vi "to_json.vi"(8 "error in":errorcluster, 11 "filterTypes in":refnum<class "filterTypes.lvclass">) -> (0 "error out":errorcluster, 2 "json":string, 3 "filterTypes out":refnum<class "filterTypes.lvclass">, 4 "Not Default":bool)   [LabVIEW 2020, in "nominal types.lvlib" / "channelFilter.lvlib" / "filterTypes.lvclass"]
uses:
  filterTypes.lvclass
  filterTypes.lvclass/filterTypes.ctl
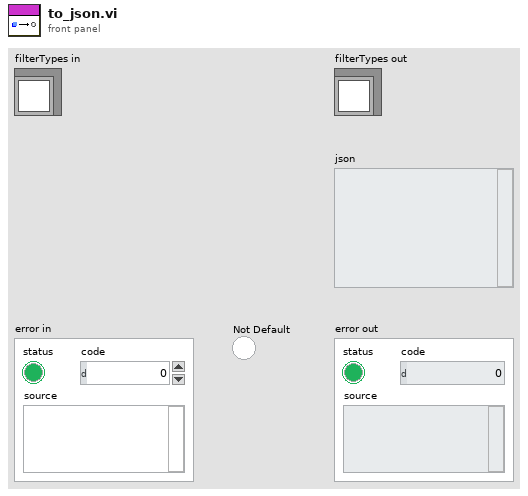
[diagram p1: front panel]
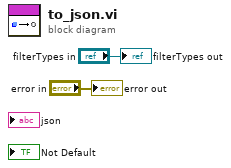
[diagram p0: block diagram]
diagram:
  "filterTypes out" <- "filterTypes in"
  "error out" <- "error in"
